vi "Simul-Progress.vi"() -> ()   [LabVIEW 2014]
uses:
  MapaIntensidade-FROG Folder14/FROG-GlobalVar.vi
panel:
  in  "milliseconds to wait":u32=5000
  out "Progresso":i32
  in  "Numero Linhas":i32=10
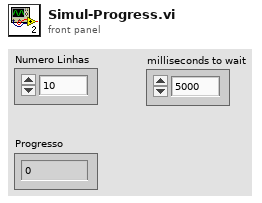
[diagram p1: front panel]
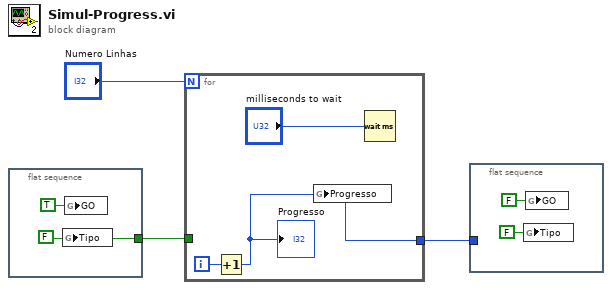
[diagram p0: block diagram]
diagram:
  n1 = flat-sequence {
    tunnel: [w4] -> w3
    frame #0 {
      w4 = FALSE ("Tipo")
      n2 = global write "FROG-GlobalVar.vi" "Tipo"(w4) -> ()
      n3 = global write "FROG-GlobalVar.vi" "GO"(TRUE ("GO")) -> ()
    }
  }
  n4 = for {
    N: "Numero Linhas" -> [_]
    tunnel: w3 -> [_]
    tunnel: [w6] -> w2
    i -> [w7]
    n5 = Increment(x=w7) -> (x+1=w6:i32)
    "Progresso" <- w6
    n6 = global write "FROG-GlobalVar.vi" "Progresso"(w6) -> ()
    n7 = Wait (ms)(milliseconds to wait="milliseconds to wait") -> ()  [unwired: 1 out]
  }
  n8 = flat-sequence {
    tunnel: w2 -> [_]
    frame #0 {
      n9 = global write "FROG-GlobalVar.vi" "Tipo"(FALSE ("Tipo")) -> ()
      n10 = global write "FROG-GlobalVar.vi" "GO"(FALSE ("GO")) -> ()
    }
  }
